vi "Strafe For Yellow.vi"   [LabVIEW 2014]
types:
  T1 = cluster{"Distance":dbl, "Rate":dbl, "Direction":bool, "Stopped":bool}[]
  T2 = cluster{"Distance":dbl, "Rate":dbl, "Direction":bool, "Stopped":bool}
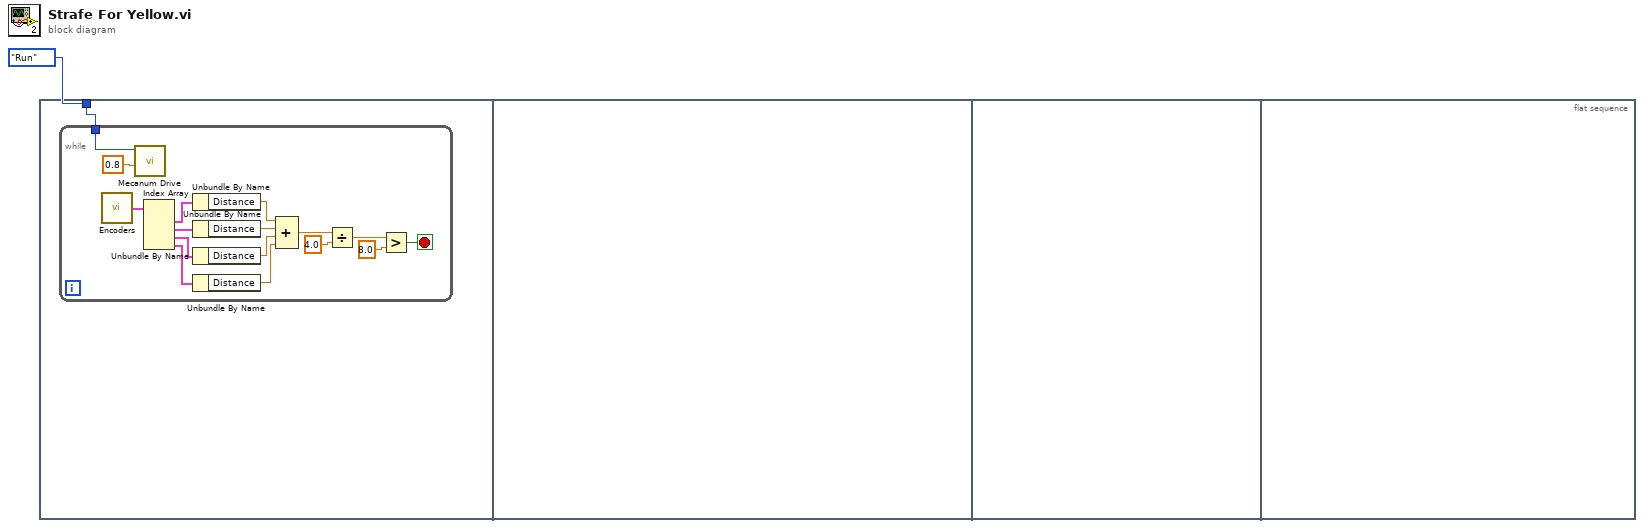
[diagram p0: block diagram]
diagram:
  n1 = flat-sequence {
    tunnel: enum8{"Start", "Run", "Finish"}."Run" ("Mode") -> [w2]
    frame #0 {
      n2 = while {
        tunnel: w2 -> [w18]
        stop <- w3 stop-if-true
        n3 = call "Encoders.vi"() -> ("Encoder"=w16:T1)  [unwired: 4 in]
        n4 = call "Mecanum Drive.vi"("Strafe"=0.8, "Mode"=w18) -> ()  [unwired: 10 in]
        n5 = Index Array(array=w16) -> (element #1=w15:T2, element #2=w14:T2, element #3=w13:T2, element #4=w12:T2)  [unwired: 4 in]
        n6 = Unbundle By Name(w15) -> ("Distance"=w11:dbl)
        n7 = Unbundle By Name(w14) -> ("Distance"=w10:dbl)
        n8 = Unbundle By Name(w13) -> ("Distance"=w9:dbl)
        n9 = Unbundle By Name(w12) -> ("Distance"=w8:dbl)
        n10 = Compound Arithmetic op=ADD(w11, w10, w9, w8) -> (w7:dbl)
        n11 = Divide(x=w7, y=4.0) -> (x/y=w5:dbl)
        n12 = Greater?(x=w5, y=8.0) -> (0:w3:bool)
      }
    }
    frame #1 {
    }
    frame #2 {
    }
    frame #3 {
    }
  }
